vi "Stop Core.vi"(10 "final error code":i32, 11 "Controller in":refnum<class "Controller.lvclass">) -> (3 "Controller out":refnum<class "Controller.lvclass">)   [LabVIEW 2019, in "Controller.lvlib" / "Controller.lvclass"]
doc: "(<B>Filename</B>: Actor Framework.lvlib:Actor.lvclass:Stop Core.vi)\n\nDefines what the actor does before it stops. Use the <B>final error code</B> input to determine whether the actor shut down in response to an error.\n\nBy default, this method passes the Stop message along to all auto-stop nested actors. A descendant class may override this method to define additional behavior, such as shutting down any processes the actor initiated in its override of the Actor Core method."
uses:
  Controller.lvclass
  Controller.lvclass/Controller.ctl
  <vilib>/ActorFramework/Actor/Actor.lvclass
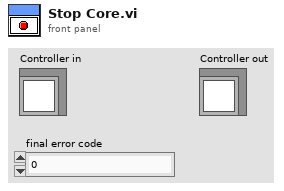
[diagram p1: front panel]
types:
  T1 = typedef "Muon Detector.lvclass/Event.ctl" = cluster{"Event Count":i32, "Device Timestamp (ms)":i32, "PC Timestamp":timestamp, "ADC Count":i32, "Event Type":u8}
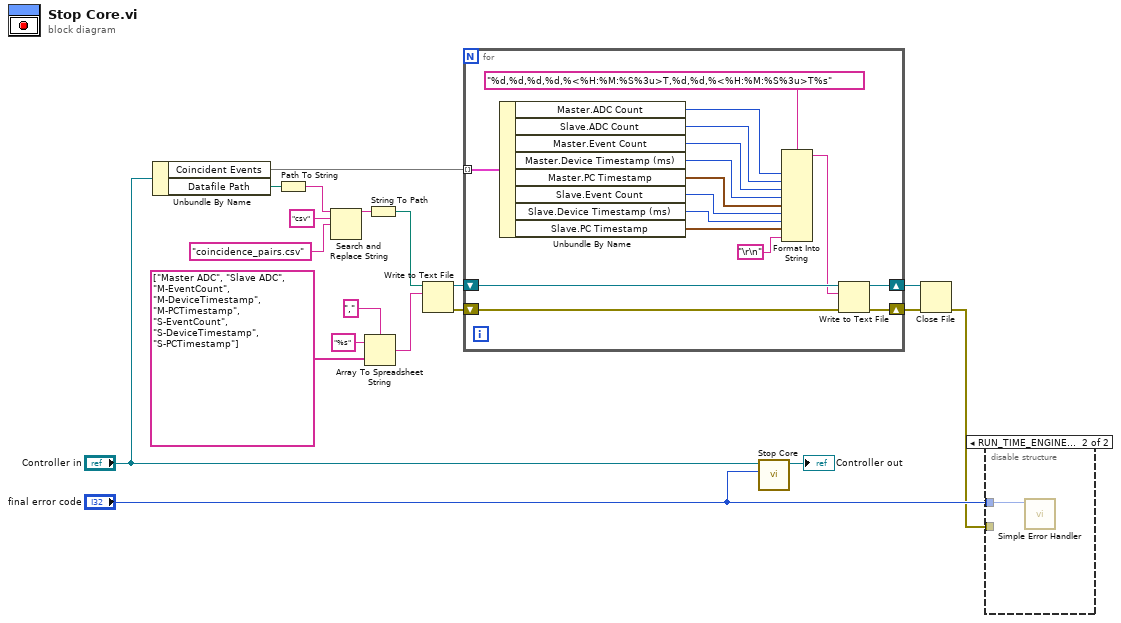
[diagram p0: block diagram]
diagram:
  n1 = Unbundle By Name("Controller in") -> ("Coincident Events"=w9:set{cluster{"Master":T1, "Slave":T1}}, "Datafile Path"=w14:path)
  n2 = Path To String(path=w14) -> (string=w17:string)
  n3 = Search and Replace String(input string=w17, search string="csv" ("substring (\"\")"), replace string="coincidence_pairs.csv" ("replace string (\"\")")) -> (result string=w13:string)  [unwired: 5 in, 3 out]
  n4 = Array To Spreadsheet String(delimiter (Tab)=",", array=string[] ["Master ADC", "Slave ADC", "M-EventCount", "M-DeviceTimestamp", "M-PCTimestamp", "S-EventCount", "S-DeviceTimestamp", "S-PCTimestamp"], 3:"%s" ("format string")) -> (spreadsheet string=w1:string)
  n5 = String To Path(string=w13) -> (path=w12:path)
  n6 = Write to Text File(file (use dialog)=w12, text=w1) -> (refnum out=w7:refnum<file>, error out=w8:errorcluster)  [unwired: 2 in, 1 out]
  n7 = for {
    tunnel: w9 -> [w35] mode=indexing
    shift-right: [w21] -> w5
    shift-left: w7 -> [w23]
    shift-right: [w22] -> w6
    shift-left: w8 -> [w24]
    n8 = Unbundle By Name(w35) -> ("Master.ADC Count"=w34:i32, "Slave.ADC Count"=w33:i32, "Master.Event Count"=w32:i32, "Master.Device Timestamp (ms)"=w31:i32, "Master.PC Timestamp"=w30:timestamp, "Slave.Event Count"=w29:i32, "Slave.Device Timestamp (ms)"=w28:i32, "Slave.PC Timestamp"=w27:timestamp)
    n9 = Format Into String(format string="%d,%d,%d,%d,%<%H:%M:%S%3u>T,%d,%d,%<%H:%M:%S%3u>T%s", w34, w33, w32, w31, w30, w29, w28, w27, "\r\n") -> (resulting string=w20:string)  [unwired: 2 in, 1 out]
    n10 = Write to Text File(file (use dialog)=w23, text=w20, error in=w24) -> (refnum out=w21:refnum<file>, error out=w22:errorcluster)  [unwired: 1 in, 1 out]
  }
  n11 = call-parent "Stop Core.vi"("final error code"="final error code", "Actor in"="Controller in") -> ("Actor out"=→"Controller out":refnum<class "Controller.lvclass">)  [unwired: 9 in]
  n12 = Close File(refnum=w5, error in=w6) -> (error out=w10:errorcluster)  [unwired: 1 out]
  n13 = disable-structure shown="RUN_TIME_ENGINE==True" {
    disable-tunnel: w10 -> [_ _]
    disable-tunnel: "final error code" -> [_ w36]
    frame condition #0 (active) {
    }
    frame condition #1 {
      n14 = call <vilib>:"Simple Error Handler.vi"("error code (no error:0)"=w36) -> ()  [unwired: 4 in, 5 out]
    }
  }
